vi "Add Expectation.vi"(8 "error in (no error)":errorcluster, 10 "Expectations":refnum<class "Expectation.lvclass">, 11 "Mock in":refnum<class "Responsive Mock.lvclass">) -> (0 "error out":errorcluster, 3 "Mock out":refnum<class "Responsive Mock.lvclass">)   [LabVIEW 2020, in "Responsive Mock.lvclass"]
uses:
  Responsive Mock.lvclass
  Expectation/Expectation.lvclass
  Responsive Mock.lvclass/Responsive Mock.ctl
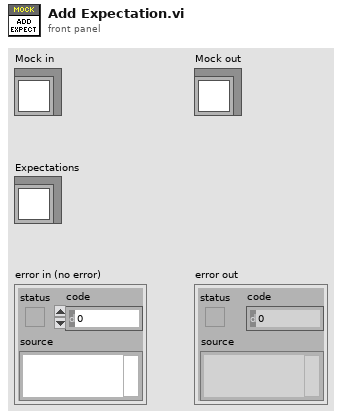
[diagram p1: front panel]
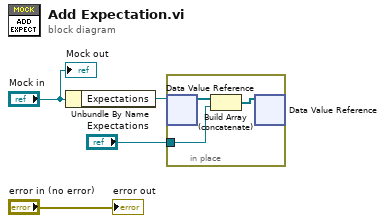
[diagram p0: block diagram]
diagram:
  n1 = Unbundle By Name("Mock in") -> ("Expectations"=w2:refnum<data-value>)
  n2 = in-place {
    in-place-border: "Expectations" -> [w6]
    n3 = in-place-dvr #1(w2) -> (w7:refnum<class "Expectation.lvclass">[])  [unwired: 1 out]
    n4 = Build Array (concatenate)(w7, w6) -> (w5:refnum<class "Expectation.lvclass">[])
    n5 = in-place-dvr #1(w5) -> ()  [unwired: 2 out]
  }
  "error out" <- "error in (no error)"
  "Mock out" <- "Mock in"
